vi "Write Command.vi"(7 "Command":T1, 8 "error in (no error)":errorcluster, 9 "Value":u8 format="%.0x", 10 "Session In":refnum<class "Session.lvclass">, 11 "Grove I2C LCD in":refnum<class "Grove I2C LCD.lvclass">) -> (0 "error out":errorcluster, 2 "Session Out":refnum<class "Session.lvclass">, 3 "Grove I2C LCD out":refnum<class "Grove I2C LCD.lvclass">)   [LabVIEW 2020, in "CTI-Peripheral.lvlib" / "Grove I2C LCD.lvclass"]
uses:
  Grove I2C LCD.lvclass
  HD44780 LCD/Command.ctl
  CTI/Session/Session.lvclass
  Grove I2C LCD.lvclass/Grove I2C LCD.ctl
  CTI/I2C Peripheral/I2C Peripheral.lvclass/I2C Peripheral.ctl
  CTI/Session/I2C Write Data.vi
  CTI/I2C Peripheral/I2C Peripheral.lvclass
  HD44780 LCD/HD44780 LCD.lvlib
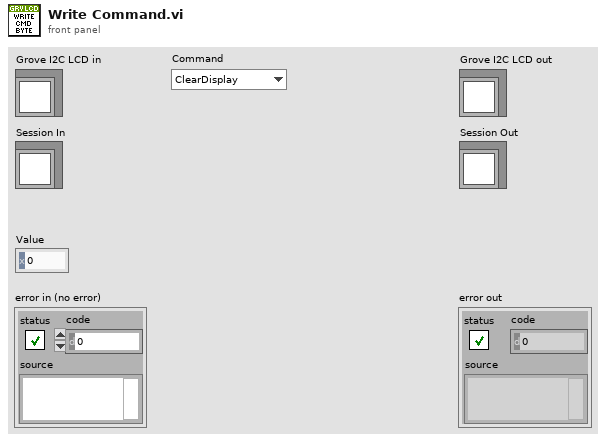
[diagram p1: front panel]
types:
  T1 = typedef "CTI-Peripheral.lvlib/HD44780 LCD.lvlib/Command.ctl" = enum16{"ClearDisplay", "ReturnHome", "EntryModeSet", "DisplayControl", "CursorShift", "FunctionSet", "SetCGRamAddr", "SetDDRamAddr"}
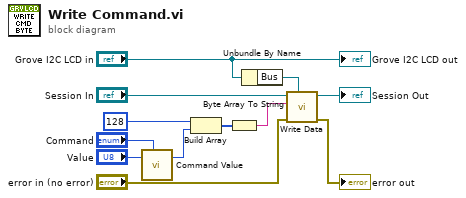
[diagram p0: block diagram]
diagram:
  n1 = call "Command Value.vi"("Value"="Value", "Command"="Command") -> ("Byte"=w5:u8)  [unwired: 5 in]
  n2 = Build Array(u8 128 ("Value"), w5) -> (w4:u8[])
  n3 = Byte Array To String(unsigned byte array=w4) -> (string=w3:string)
  n4 = Unbundle By Name("Grove I2C LCD in") -> ("Bus"=w11:refnum<class "I2C Peripheral.lvclass">)
  n5 = call "Write Data.vi"("I2C Peripheral"=w11, "error in (no error)"="error in (no error)", "Data"=w3, "Session In"="Session In") -> ("error out"=→"error out":errorcluster, "Session Out"=→"Session Out":refnum<class "Session.lvclass">)  [unwired: 6 in]
  "Grove I2C LCD out" <- "Grove I2C LCD in"
